vi "Abre pasta.vi"(0 "Pasta do ensaio":path) -> (1 "Dados":string, 2 "Infos para processamento out":T1={"Diâmetro do furo [mm]"=1.4, "Diâmetro da linha média [mm]"=5.0, "IncF"=0.2, "Módulo de elasticidade [GPa]"=207.0, "Módulo de Poisson"=0.3, "Tipo de roseta utilizada"=enum."Tipo A", "Método de análise"=enum."Simplificado 2008", "Pfinal"=0.3, "Parar auto."=TRUE})   [LabVIEW 2016]
uses:
  Controles/Infos para processamento.ctl
panel:
  in  "Confirmar dados":bool
  # "Estes foram os dados encontrados no arquivo de informações. Eles estão corretos?"
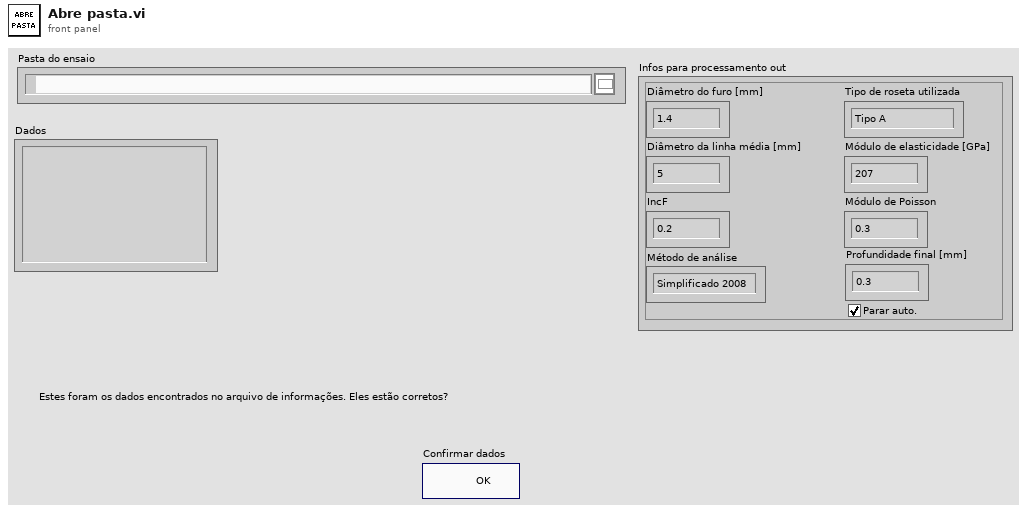
[diagram p1: front panel]
types:
  T1 = typedef "Infos para processamento.ctl" = cluster{"Diâmetro do furo [mm]":dbl, "Diâmetro da linha média [mm]":dbl, "IncF":dbl, "Módulo de elasticidade [GPa]":dbl, "Módulo de Poisson":dbl, "Tipo de roseta utilizada":enum16{"Tipo A", "Tipo B", "Tipo C"}, "Método de análise":enum16{"Não uniforme 2013", "Simplificado 2013", "Simplificado 2008"}, "Pfinal":dbl, "Parar auto.":bool}
  T2 = enum16{"Não uniforme 2013", "Simplificado 2013", "Simplificado 2008"}
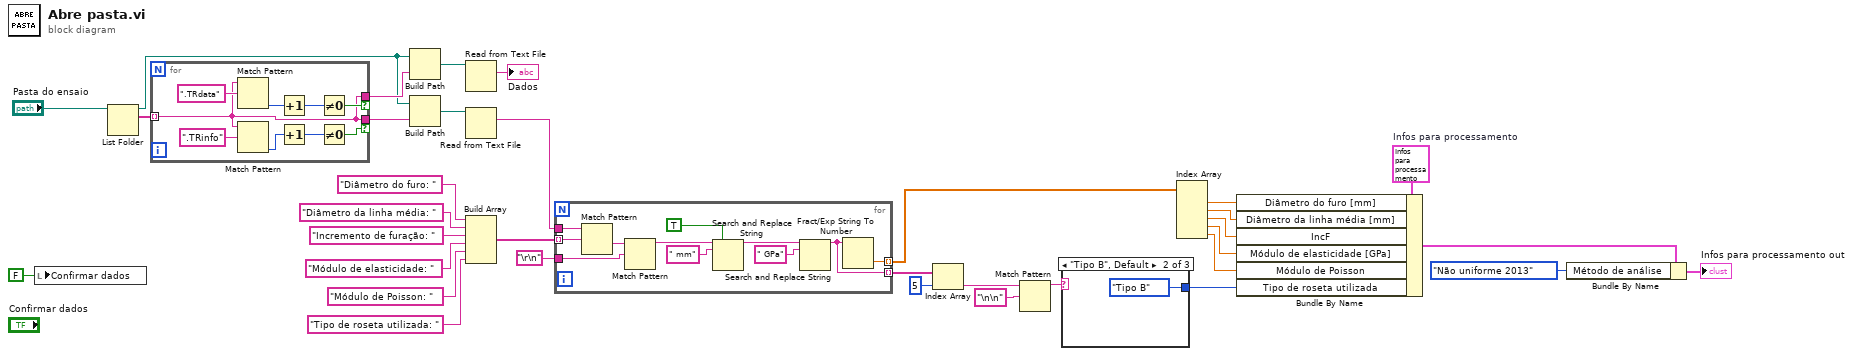
[diagram p0: block diagram]
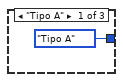
[diagram p2: hidden frame]
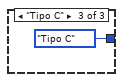
[diagram p3: hidden frame]
diagram:
  w17 = T1 {"Diâmetro do furo [mm]"=1.4, "Diâmetro da linha média [mm]"=5.0, "IncF"=0.2, "Módulo de elasticidade [GPa]"=207.0, "Módulo de Poisson"=0.3, "Tipo de roseta utilizada"=enum."Tipo A", "Método de análise"=enum."Simplificado 2008", "Pfinal"=0.3, "Parar auto."=TRUE}  # Infos para processamento
  n1 = local write "Confirmar dados"(FALSE ("Confirmar dados")) -> ()
  n2 = List Folder(path="Pasta do ensaio") -> (path out=w29:path, filenames=w33:string[])  [unwired: 3 in, 2 out]
  n3 = for {
    tunnel: w33 -> [w35] mode=indexing
    tunnel: [w35] -> w32 if=w39
    tunnel: [w35] -> w28 if=w36
    n4 = Match Pattern(string=w35, regular expression=".TRdata") -> (offset past match=w41:i32)  [unwired: 1 in, 3 out]
    n5 = Match Pattern(string=w35, regular expression=".TRinfo") -> (offset past match=w37:i32)  [unwired: 1 in, 3 out]
    n6 = Increment(x=w41) -> (x+1=w40:i32)
    n7 = Increment(x=w37) -> (x+1=w38:i32)
    n8 = Not Equal To 0?(x=w40) -> (x != 0?=w39:bool)
    n9 = Not Equal To 0?(x=w38) -> (x != 0?=w36:bool)
  }
  n10 = Build Path(base path=w29, name or relative path=w32) -> (appended path=w31:path)
  n11 = Build Path(base path=w29, name or relative path=w28) -> (appended path=w30:path)
  n12 = Read from Text File(file (use dialog)=w31) -> (text=→"Dados":string)  [unwired: 3 in, 3 out]
  n13 = Read from Text File(file (use dialog)=w30) -> (text=w20:string)  [unwired: 3 in, 3 out]
  n14 = Build Array("Diâmetro do furo: " ("string"), "Diâmetro da linha média: " ("string"), "Incremento de furação: " ("string"), "Módulo de elasticidade: " ("string"), "Módulo de Poisson: " ("string"), "Tipo de roseta utilizada: " ("string")) -> (w19:string[])
  n15 = for {
    tunnel: w20 -> [w54]
    tunnel: w19 -> [w53] mode=indexing
    tunnel: "\r\n" -> [w51]
    tunnel: [w45] -> w16 mode=indexing
    tunnel: [w44] -> w15 mode=indexing
    n16 = Match Pattern(string=w54, regular expression=w53) -> (after substring=w52:string)  [unwired: 1 in, 3 out]
    n17 = Match Pattern(string=w52, regular expression=w51) -> (before substring=w50:string)  [unwired: 1 in, 3 out]
    n18 = Search and Replace String(replace all?=TRUE ("replace all? (F)"), input string=w50, search string=" mm") -> (result string=w46:string)  [unwired: 5 in, 3 out]
    n19 = Search and Replace String(input string=w46, search string=" GPa") -> (result string=w45:string)  [unwired: 6 in, 3 out]
    n20 = Fract/Exp String To Number(string=w45) -> (number=w44:dbl)  [unwired: 3 in, 1 out]
  }
  n21 = Index Array(array=w16, index=5) -> (element=w7:string)
  n22 = Match Pattern(string=w7, regular expression="\n\n") -> (before substring=w6:string)  [unwired: 1 in, 3 out]
  n23 = case shown="\"Tipo B\", Default" w6 {
    tunnel: [enum16{"Tipo A", "Tipo B", "Tipo C"}."Tipo A" ("Tipo de roseta utilizada") enum16{"Tipo A", "Tipo B", "Tipo C"}."Tipo B" ("Tipo de roseta utilizada") enum16{"Tipo A", "Tipo B", "Tipo C"}."Tipo C" ("Tipo de roseta utilizada")] -> w8
    frame "Tipo A" {
    }
    frame "Tipo B", Default {
    }
    frame "Tipo C" {
    }
  }
  n24 = Index Array(array=w15) -> (element #1=w14:dbl, element #2=w13:dbl, element #3=w12:dbl, element #4=w11:dbl, element #5=w10:dbl)  [unwired: 5 in]
  n25 = Bundle By Name(cluster=w17, "Diâmetro do furo [mm]"=w14, "Diâmetro da linha média [mm]"=w13, "IncF"=w12, "Módulo de elasticidade [GPa]"=w11, "Módulo de Poisson"=w10, "Tipo de roseta utilizada"=w8) -> (w1:T1)
  n26 = Bundle By Name(cluster=w1, "Método de análise"=T2."Não uniforme 2013") -> (→"Infos para processamento out":T1)
